vi "Time units.vi"(9 "Array":dbl[](array[numeric]), 10 "Numeric":dbl format="%#_8f") -> (1 "Scaled Array":dbl[](array[numeric]), 2 "Scaled Number":dbl, 3 "modified unit":string)   [LabVIEW 2012, in "Design Server.lvlib"]
uses:
  Design Server.lvlib
panel:
  out "x^y":dbl
  out "logx(y)":dbl
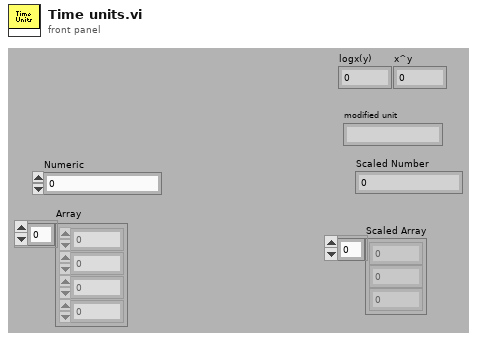
[diagram p1: front panel]
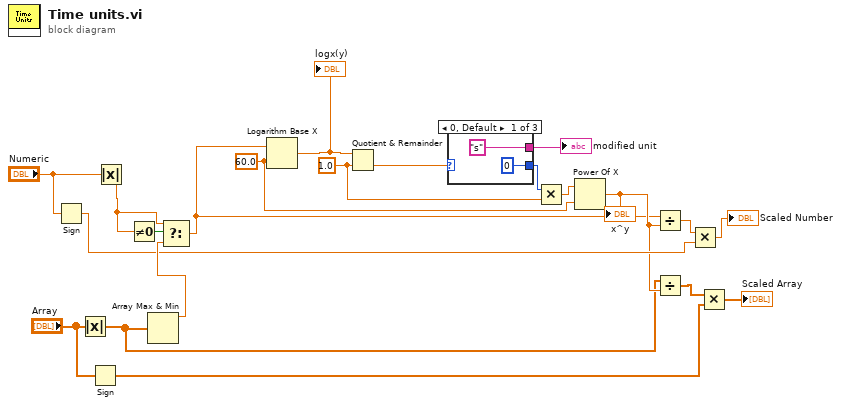
[diagram p0: block diagram]
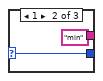
[diagram p2: hidden frame]
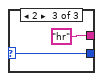
[diagram p3: hidden frame]
diagram:
  w4 = 60.0 ("x")
  w21 = 1.0 ("y")
  n1 = Sign(1:"Numeric") -> (0:w13:dbl)
  n2 = Absolute Value(x="Array") -> (abs(x)=w7:dbl[])
  n3 = Sign(1:"Array") -> (0:w12:dbl[])
  n4 = Absolute Value(x="Numeric") -> (abs(x)=w16:dbl)
  n5 = Not Equal To 0?(x=w16) -> (x != 0?=w18:bool)
  n6 = Array Max & Min(array=w7) -> (max value=w17:dbl)  [unwired: 3 out]
  n7 = Select(t=w16, s=w18, f=w17) -> (s? t:f=w6:dbl)
  n8 = Logarithm Base X(1:w4, 2:w6) -> (0:w5:dbl)
  "logx(y)" <- w5
  n9 = Quotient & Remainder(x=w5, y=w21) -> (floor(x/y)=w20:dbl)  [unwired: 1 out]
  n10 = case shown="0, Default" w20 {
    selector: w20 -> [_ w24 w26]
    tunnel: ["s" "min" "hr"] -> w1
    tunnel: [0 w24 w26] -> w19
    frame 0, Default {
    }
    frame 1 {
    }
    frame 2 {
    }
  }
  "modified unit" <- w1
  n11 = Multiply(x=w19, y=w21) -> (x*y=w3:dbl)
  n12 = Power Of X(1:w4, 2:w3) -> (0:w8:dbl)
  "x^y" <- w8
  n13 = Divide(x=w6, y=w8) -> (x/y=w10:dbl)
  n14 = Divide(x=w7, y=w8) -> (x/y=w9:dbl[])
  n15 = Multiply(x=w10, y=w13) -> (x*y=→"Scaled Number":dbl)
  n16 = Multiply(x=w9, y=w12) -> (x*y=→"Scaled Array":dbl[])
